vi "Do.vi"(8 "error in":errorcluster, 10 "Actor in":refnum<class "Actor.lvclass">, 11 "Change Filter State":refnum<class "Change Filter State.lvclass">) -> (0 "error out":errorcluster, 2 "Actor out":refnum<class "Actor.lvclass">)   [LabVIEW 2014, in "Controller.lvlib" / "Change Filter State.lvclass"]
doc: "(<B>Filename</B>: Actor Framework.lvlib:Message.lvclass:Do.vi)\n\nDefines what a message does when it is received by an actor. Generally, a message instructs an actor to invoke one of its methods. By default, this method does nothing. A child class must override it to define behavior. Create a child class by using the Actor Framework Message Maker dialog box."
uses:
  Change Filter State.lvclass
  <vilib>/ActorFramework/Actor/Actor.lvclass
  Controller.lvclass
  Update Switch State MSG/Update Switch MSG.lvclass/Update Switch MSG.ctl
  SuperActor/Ex Nested.lvclass/Ex Nested.ctl
  Controller.lvclass/Controller.ctl
  <vilib>/DAQmx/write.llb/DAQmx Write (Digital 1D Bool NChan 1Samp 1Line).vi
  Update Switch State MSG/Read SwitchState.vi
  SuperActor/Read CVT Session.vi
  SuperActor/Read Log Session.vi
  Accessors/Read Filter Task.vi
  Accessors/Read Switch DVR.vi
  <vilib>/DAQmx/miscellaneous.llb/DAQmx Fill In Error Info.vi
  reusable/Switch/Switch.lvclass
  <userlib>/_Session Fwk/Session - Root.lvclass
  reusable/Session APIs/Session Log/System Log.lvclass
  reusable/Session APIs/CVT/CVT.lvclass
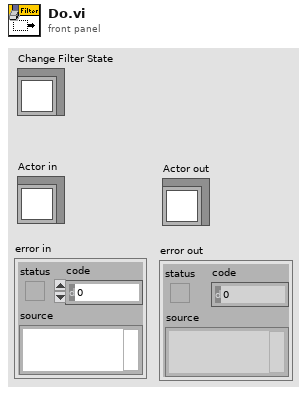
[diagram p1: front panel]
types:
  T1 = typedef "Session - Root.lvclass/Session Handle.ctl" = refnum<data-value>
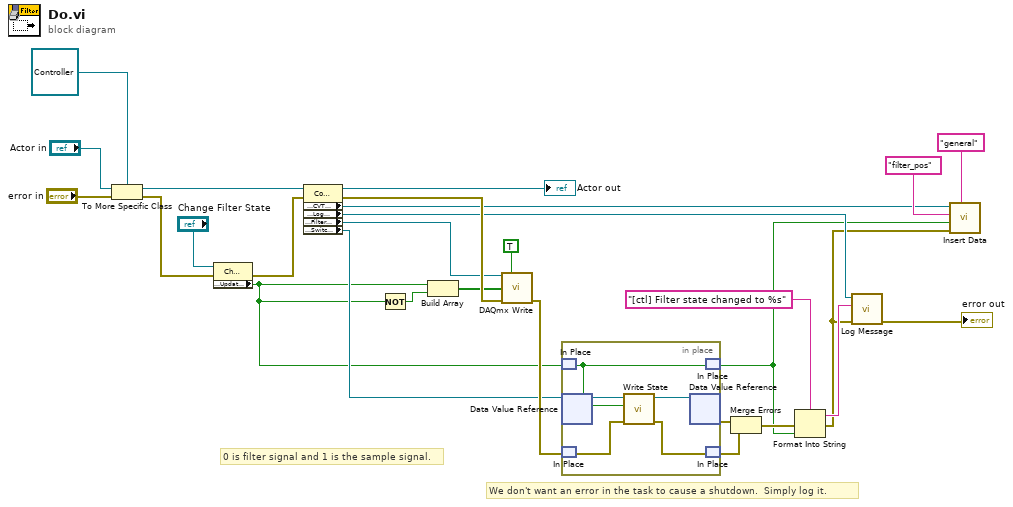
[diagram p0: block diagram]
diagram:
  # "0 is filter signal and 1 is the sample signal."
  # "We don't want an error in the task to cause a shutdown.  Simply log it."
  n1 = To More Specific Class(target class=refnum<class "Controller.lvclass"> refnum ("Controller in"), reference="Actor in", error in="error in") -> (specific class reference=w6:refnum<class "Controller.lvclass">, error out=w4:errorcluster)
  n2 = property class="Change Filter State MSG"(reference="Change Filter State", error in=w4) -> (error out=w1:errorcluster, "Accessors:UpdateSw"=w5:bool)  [unwired: 1 out]
  n3 = property class="Controller"(reference=w6, error in=w1) -> (reference out=→"Actor out":refnum<class "Controller.lvclass">, error out=w20:errorcluster, "Accessors:CVT Session"=w14:T1, "Accessors:Log Session"=w15:T1, "Accessors:Filter Task"=w7:refnum<k21>, "Accessors:Switch DVR"=w8:refnum<data-value>)
  n4 = Not(x=w5) -> (.not. x?=w19:bool)
  n5 = Build Array(w5, w19) -> (w18:bool[])
  n6 = call-poly <vilib>:"DAQmx Write.vi"("task/channels in"=w7, "auto start"=TRUE, "data"=w18, "error in"=w20) -> ("error out"=w12:errorcluster)  [unwired: 9 in, 2 out]
  n7 = in-place {
    n8 = in-place-match #1(w5) -> (w29:bool)
    n9 = in-place-dvr #2(w8) -> (w33:refnum<class "Switch.lvclass">)  [unwired: 1 out]
    n10 = in-place-match #3(w12) -> (w30:errorcluster)
    n11 = call-dynamic "Write State.vi"("error in"=w30, "State"=w29, "Switch in"=w33) -> ("error out"=w31:errorcluster, "Switch out"=w32:refnum<class "Switch.lvclass">)  [unwired: 7 in]
    n12 = in-place-dvr #2(w32) -> (w24:errorcluster)  [unwired: 1 out]
    n13 = in-place-match #1(w29) -> (w9:bool)
    n14 = in-place-match #3(w31) -> (w13:errorcluster)
  }
  n15 = Merge Errors(w24, w13) -> (w11:errorcluster)
  n16 = Format Into String(format string="[ctl] Filter state changed to %s" ("MSG In"), error in=w11, w9) -> (resulting string=w21:string, error out=w10:errorcluster)  [unwired: 1 in]
  n17 = call "Log Message.vi"("error in"=w10, "MSG In"=w21, "session in"=w15) -> ("error out"=→"error out":errorcluster)  [unwired: 7 in, 1 out]
  n18 = call "Insert Data.vi"("Group"="general", "error in"=w10, "Data"=w9, "tag"="filter_pos", "CVT Session In"=w14) -> ()  [unwired: 5 in, 2 out]
